vi "WLAN Two Site Example_Remote PC.vi"(5 "Single DUT Mode?":bool, 7 "Stop if fail":bool, 9 "Select Test Item (TX Verification)":T1={"Tx_ 802.11a/g OFDM"=TRUE, "Tx_ 802.11b DSSS/CCK"=FALSE, "Tx_ 802.11n OFDM "=TRUE, "Tx_ 802.11ac OFDM "=TRUE}, 10 "Select Test Content":T3, 11 "SET RUN TIMES":i32=1) -> (1 "Results":T2, 2 "Total test time":dbl=137.063, 3 "RUN TIMES":i32=1)   [LabVIEW 2012]
uses:
  WLAN SubVIs/WLAN Autotest Library/niWLAN/WLAN -  niWLAN - INC - Select Measurement.ctl
  System SubVIs/Select_Test_Content.ctl
  Report SubVIs/TypeDef/Report Log Flow Control.ctl
  Report SubVIs/TypeDef/DUT Number.ctl
  WLAN SubVIs/WLAN Autotest Library/TestExample/QCA/WB335B/TypeDef/WLAN Flow Control.ctl
  System SubVIs/Ctl_Ant_Number.ctl
  Remote Sever SubVIs/TypeDef/Send Command Message.ctl
panel:
  in  "Select Test Item (TX Verification) 2":T1={"Tx_ 802.11a/g OFDM"=TRUE, "Tx_ 802.11b DSSS/CCK"=FALSE, "Tx_ 802.11n OFDM "=TRUE, "Tx_ 802.11ac OFDM "=TRUE}
  out "RUN TIMES 2":i32=1
  out "MAC&SN 3":string
  out "Results 2":T2
  out "MAC&SN 2":string
  out "MAC&SN":string
  out "DUT2 log path":path
  out "DUT1 log path":path
  in  "Tab Control":T4(tab)
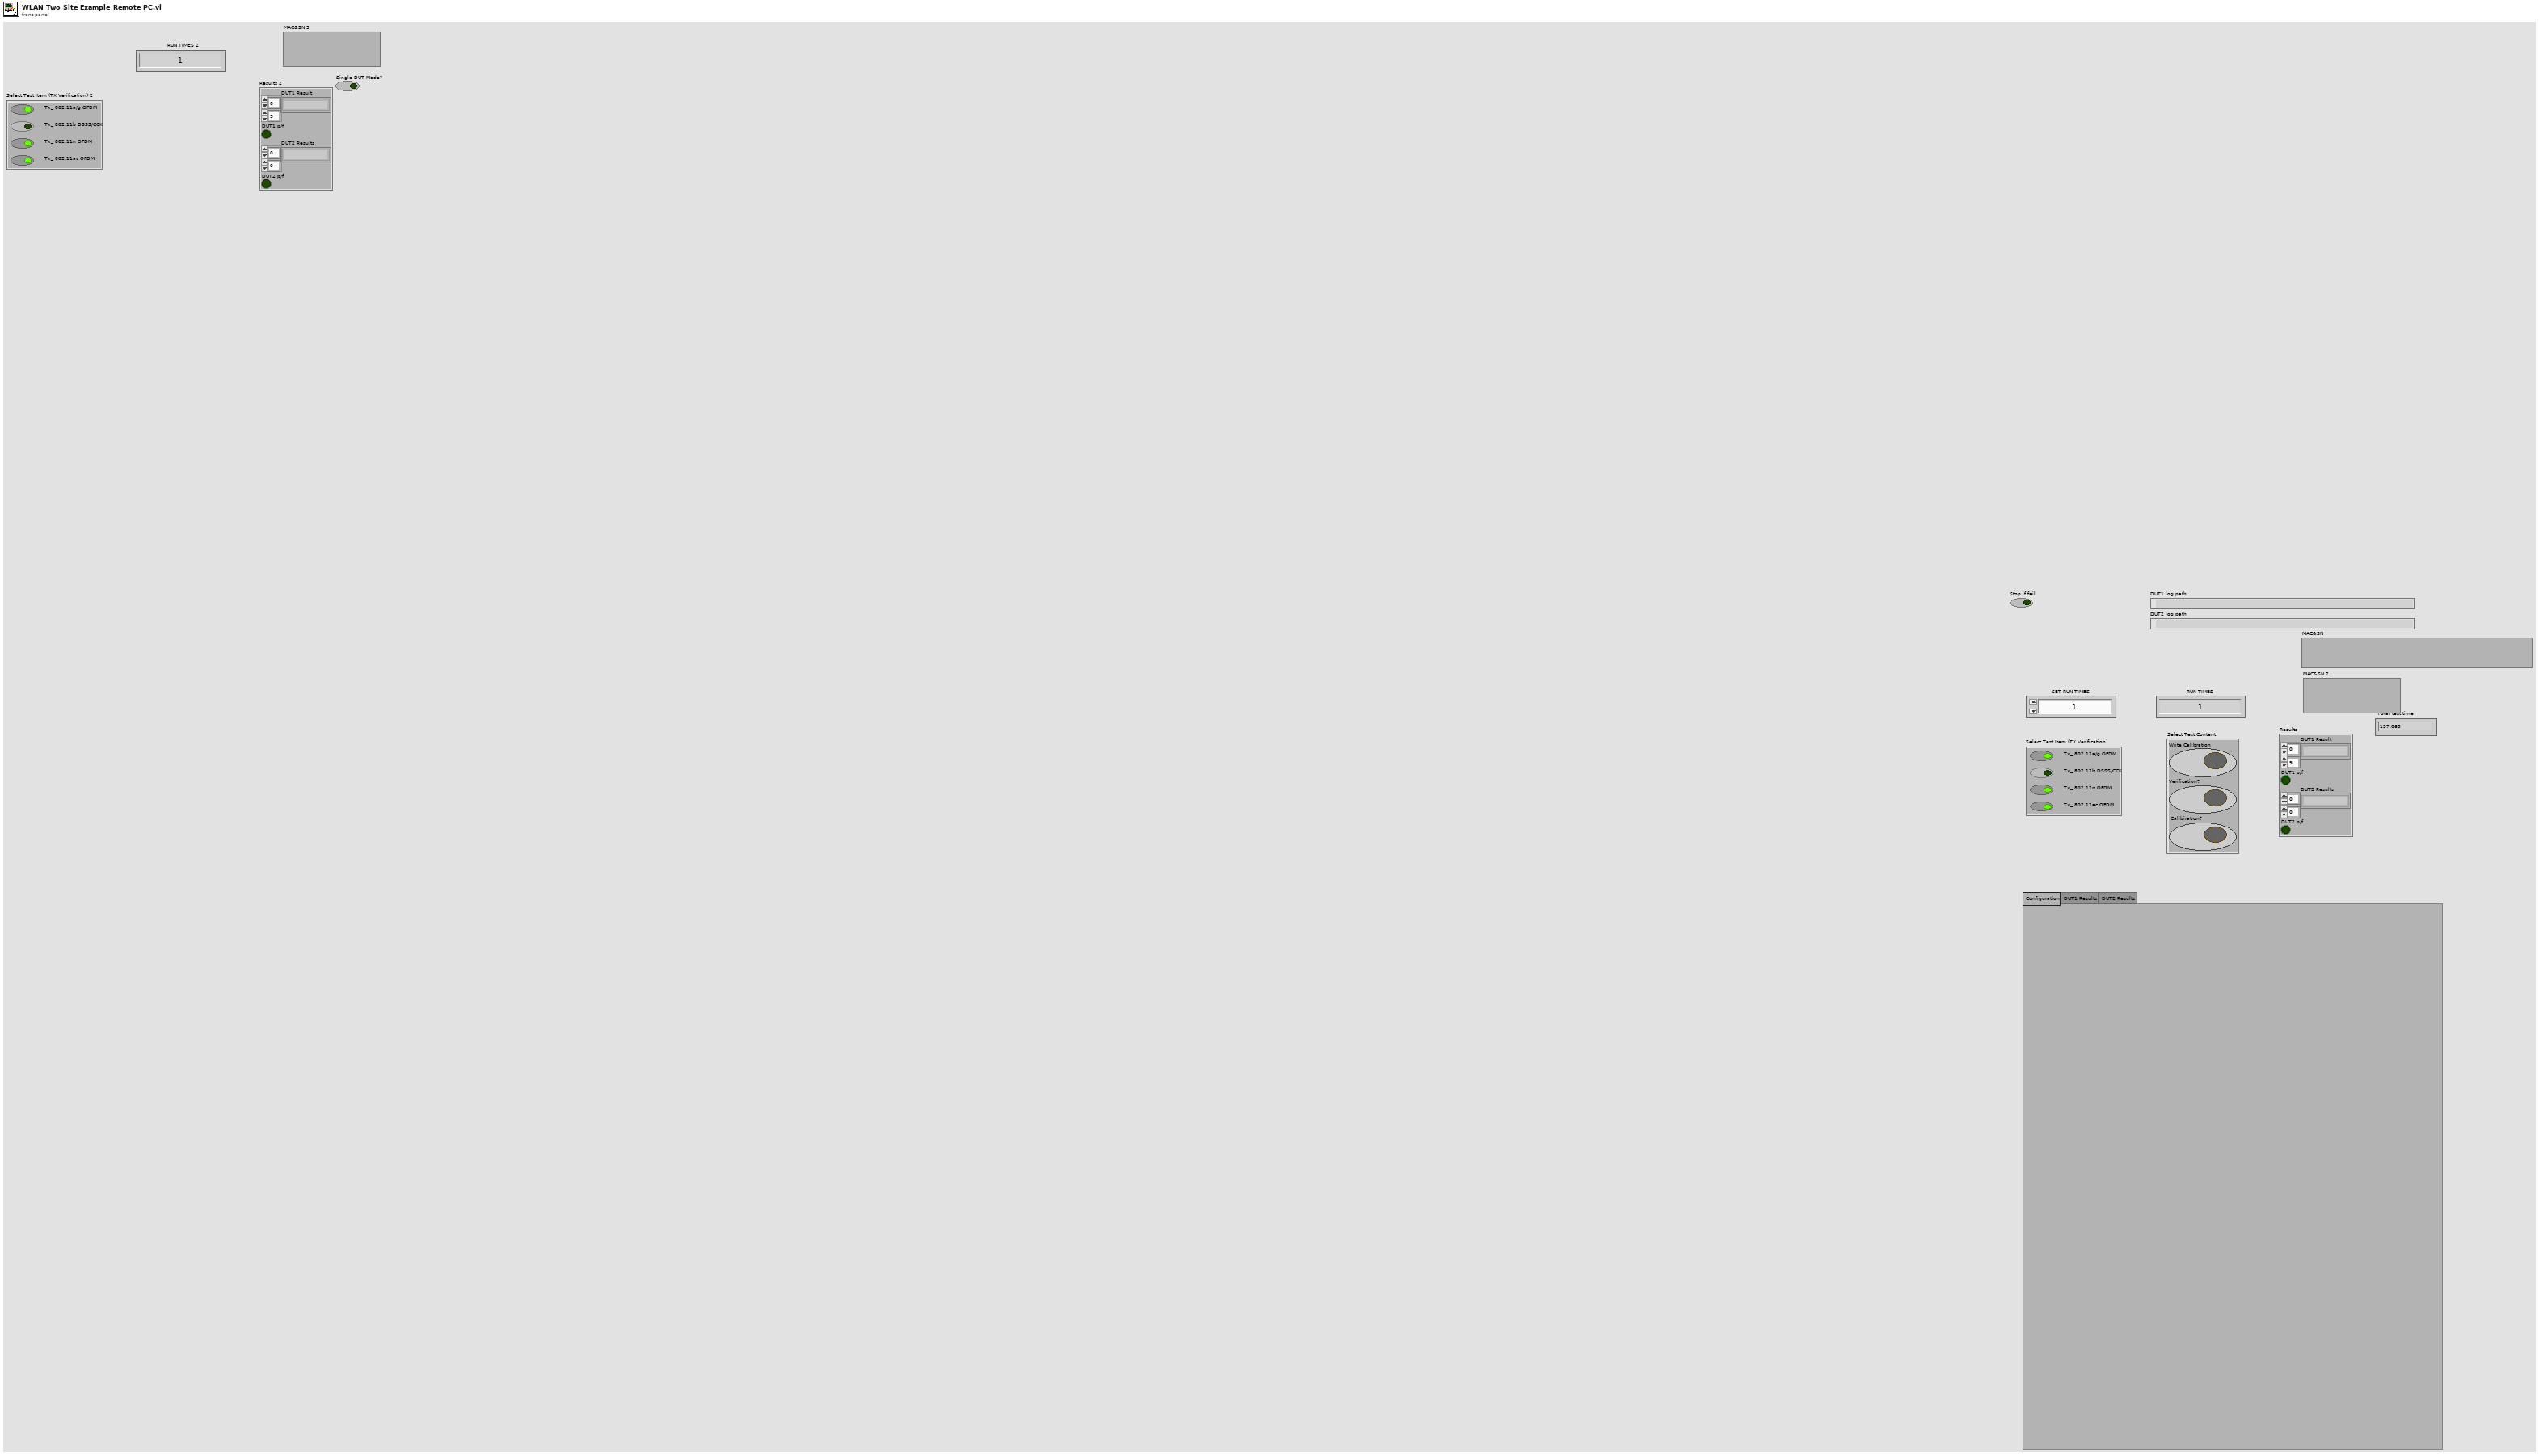
[diagram p1: front panel]
types:
  T1 = typedef "WLAN -  niWLAN - INC - Select Measurement.ctl" = cluster{"Tx_ 802.11a/g OFDM":bool, "Tx_ 802.11b DSSS/CCK":bool, "Tx_ 802.11n OFDM ":bool, "Tx_ 802.11ac OFDM ":bool}
  T2 = cluster{"DUT1 Result":string[][], "DUT1 p/f":bool, "DUT2 Results":string[][], "DUT2 p/f":bool}
  T3 = typedef "Select_Test_Content.ctl" = cluster{"Write Calibration":bool, "Verification?":bool, " Calibiration?":bool}
  T4 = enum32{"Configuration", "DUT1 Results", "DUT2 Results "}
  T5 = typedef "DUT Number.ctl" = string
  T6 = typedef "Report Log Flow Control.ctl" = enum16{"Create Log File", "Append Test Item Head", "Append WLAN TX IQ Result", "Append WLAN TX Spectrum Result", "Append WLAN RX Result", "Append BT TX BR Result", "Append BT TX EDR Result", "Append Customized Text", "Append BT RX Result", "Read Log File", "Save Test Time"}
  T7 = typedef "WLAN Flow Control.ctl" = enum16{"Initial WLAN DUT", "Load WLAN DUT Only", "Close WLAN Test", "Power Calibration", "TX Verification", "RX Verification", "Write Memory"}
  T8 = typedef "Send Command Message.ctl" = string
  T9 = typedef "Ctl_Ant_Number.ctl" = enum16{"1", "2", "3"}
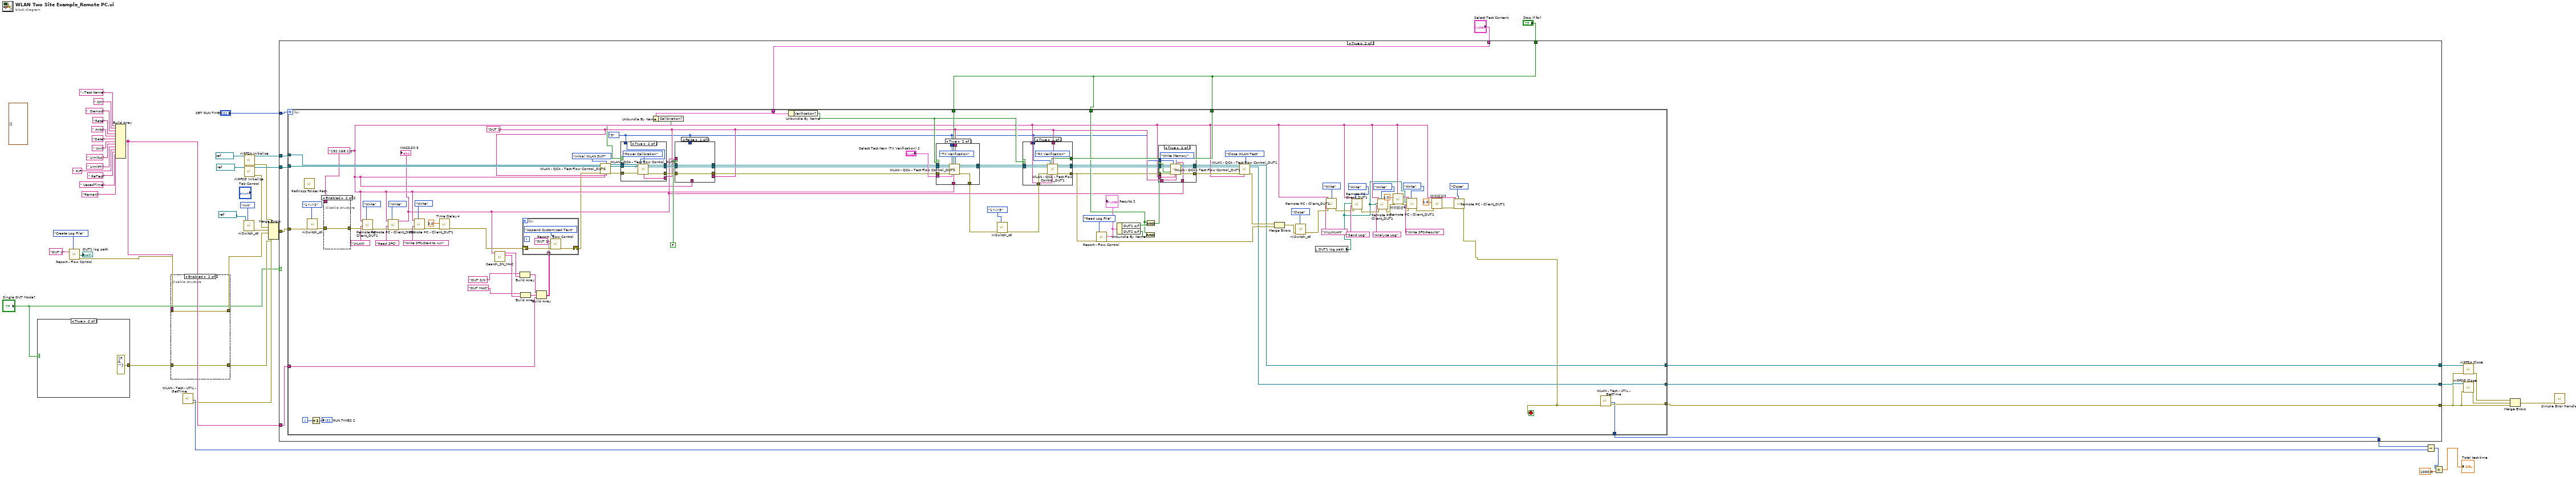
[diagram p0: block diagram]
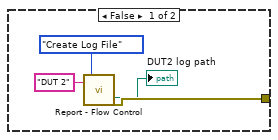
[diagram p2: hidden frame]
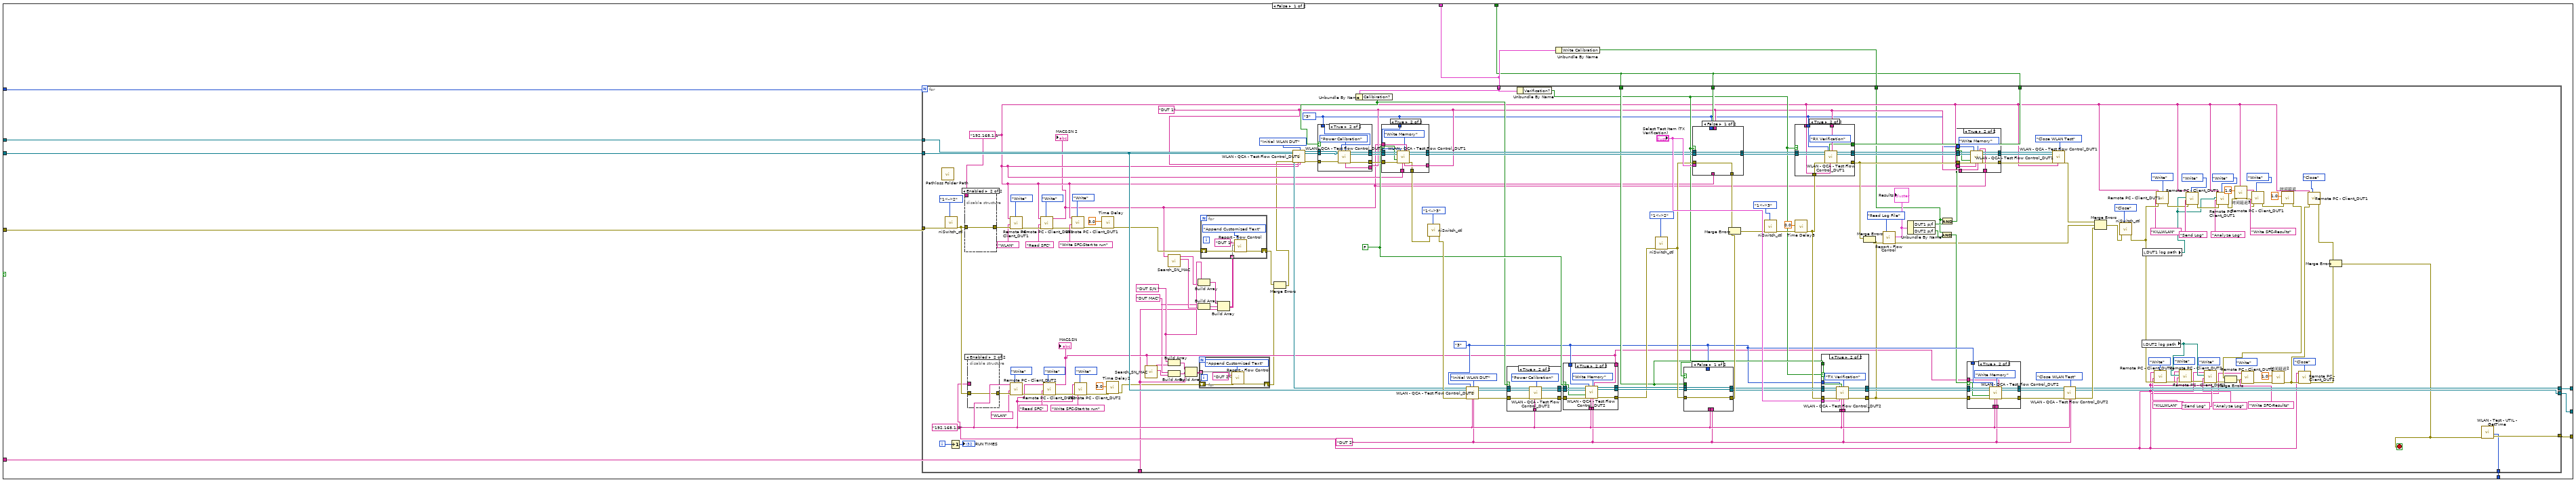
[diagram p3: hidden frame]
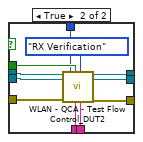
[diagram p7: hidden frame]
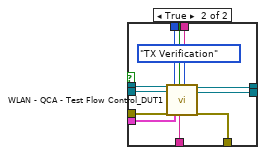
[diagram p10: hidden frame]
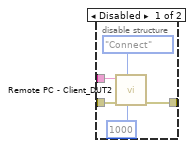
[diagram p12: hidden frame]
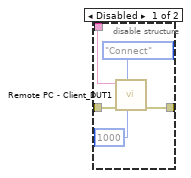
[diagram p13: hidden frame]
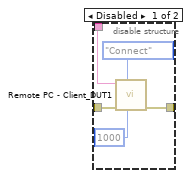
[diagram p20: hidden frame]
diagram:
  (unwired) cluster{u32, u32, u32, u32, u32, u32}[] [] ("History Data")
  n1 = case shown="True" "Single DUT Mode?" {
    tunnel: [w49 errorcluster {"status"=FALSE, "code"=0, "source"=""} ("error out")] -> w19
    frame False {
      n2 = call "Report - Flow Control.vi"("DUT Number (Each Control)"=T5 "DUT 2", "Reprot Log Flow Control"=Report_Log_Flow_Control."Create Log File") -> ("DUT2 log path"=→"DUT2 log path":path, "error out"=w49:errorcluster)  [unwired: 12 in, 4 out]
    }
    frame True {
    }
  }
  n3 = call "Report - Flow Control.vi"("DUT Number (Each Control)"=T5 "DUT 1", "Reprot Log Flow Control"=Report_Log_Flow_Control."Create Log File") -> ("DUT1 log path"=→"DUT1 log path":path, "error out"=w20:errorcluster)  [unwired: 12 in, 4 out]
  n4 = Build Array(";;Test Name", " CH", "  Demod", "Rate", " Ants", "Data", " Unit", " LimitLo", " LimitHi", " P/F", " ReTest", " UesedTime", "Remark" ("元素")) -> (w6:string[])
  n5 = disable-structure shown="Enabled" {
    disable-tunnel: [w57 w62] -> w27
    disable-tunnel: [w56 w63] -> w26
    disable-tunnel: w20 -> [w55 w63]
    disable-tunnel: w19 -> [w54 w62]
    disable-tunnel: w6 -> [w53 _]
    frame Disabled {
      n6 = call "Report - Flow Control.vi"("DUT Number (Each Control)"=T5 "DUT 1", "Text Input"=w53, "error in"=w55, "Reprot Log Flow Control"=Report_Log_Flow_Control."Append Customized Text") -> ("error out"=w56:errorcluster)  [unwired: 10 in, 5 out]
      n7 = call "Report - Flow Control.vi"("DUT Number (Each Control)"=T5 "DUT 2", "Text Input"=w53, "error in"=w54, "Reprot Log Flow Control"=Report_Log_Flow_Control."Append Customized Text") -> ("error out"=w57:errorcluster)  [unwired: 10 in, 5 out]
    }
    frame Enabled {
    }
  }
  n8 = call "WLAN - Test - UTIL - GetTime.vi"() -> ("error out"=w31:errorcluster, "millisecond timer value"=w32:u32)  [unwired: 9 in, 1 out]
  n9 = call "niSwitch_ctl.vi"("Flow Control"=enum16{"Init", "1<->2", "1<->3", "Close"}."Init" ("Ctrl"), "Switch In"=refnum<k15> "2598" ("resource name")) -> ("error out"=w40:errorcluster)  [unwired: 7 in, 2 out]
  n10 = call <instrlib>:"niRFSA Initialize.vi"("resource name"=refnum<k15> "VST1") -> ("instrument handle"=w45:refnum<k15>, "error out"=w42:errorcluster)  [unwired: 13 in]
  n11 = call <instrlib>:"niRFSG Initialize.vi"("resource name"=refnum<k15> "VST1") -> ("instrument handle"=w44:refnum<k15>, "error out"=w41:errorcluster)  [unwired: 13 in]
  n12 = Merge Errors(w42, w41, w40, w26, w27, w31) -> (w39:errorcluster)
  n13 = case shown="True" "Single DUT Mode?" {
    tunnel: w45 -> [w75 w413]
    tunnel: w44 -> [w74 w412]
    tunnel: "SET RUN TIMES" -> [w73 w411]
    tunnel: w39 -> [w72 w414]
    tunnel: [w71 w406] -> w2
    tunnel: [w70 w405] -> w36
    tunnel: [w69 w407] -> w35
    tunnel: w6 -> [w68 w410]
    tunnel: [w67 w404] -> w5
    tunnel: "Select Test Content" -> [w65 w409]
    tunnel: "Stop if fail" -> [w64 w408]
    frame False {
      n14 = Unbundle By Name(w65) -> ("Write Calibration"=w66:bool)
      n15 = for {
        N: w73 -> [_]
        tunnel: w72 -> [w237]
        tunnel: w75 -> [w179]
        tunnel: w74 -> [w224]
        tunnel: [w193] -> w67
        tunnel: [w207] -> w71
        tunnel: [w206] -> w70
        tunnel: [w192] -> w69
        tunnel: w64 -> [w143]
        tunnel: w64 -> [w129]
        tunnel: w64 -> [w142]
        tunnel: w65 -> [w128]
        tunnel: w66 -> [w111]
        tunnel: w68 -> [w83]
        i -> [w234]
        stop <- w194 stop-if-true
        w88 = "DUT MAC" ("string")
        w89 = "DUT S/N " ("string")
        w130 = FALSE
        (unwired) enum16{"Connect", "Read", "Write", "Close"}."Write" ("Flow Contorl")
        (unwired) enum16{"Connect", "Read", "Write", "Close"}."Write" ("Flow Contorl")
        (unwired) enum16{"Connect", "Read", "Write", "Close"}."Write" ("Flow Contorl")
        w101 = Ctl_Ant_Number."3" ("Ant Number")
        w108 = Ctl_Ant_Number."3" ("Ant Number")
        w103 = "192.168.1.2" ("ART2 IP Address (\"\": localhost) (Initial)")
        w102 = "DUT 2" ("Board Name (TX RX Verification)")
        w113 = "DUT 1" ("Board Name (TX RX Verification)")
        w114 = "192.168.1.1" ("ART2 IP Address (\"\": localhost)")
        n16 = call "Pathloss Folder Path.vi"() -> ()  [unwired: 11 in, 1 out]
        n17 = call "niSwitch_ctl.vi"("Flow Control"=enum16{"Init", "1<->2", "1<->3", "Close"}."1<->2", "error in"=w237) -> ("error out"=w170:errorcluster)  [unwired: 7 in, 2 out]
        n18 = Increment(x=w234) -> (x+1=→"RUN TIMES":i32)
        n19 = disable-structure shown="Enabled" {
          disable-tunnel: [w371 w373] -> w232
          disable-tunnel: w170 -> [w369 w373]
          disable-tunnel: w114 -> [w368 _]
          frame Disabled {
            n20 = call "Remote PC - Client_DUT1.vi"("Remote Sever Port (2800)"=u16 1000, "Flow Contorl"=enum16{"Connect", "Read", "Write", "Close"}."Connect", "error in"=w369, "IP Address"=w368) -> ("error out"=w371:errorcluster)  [unwired: 5 in, 2 out]
          }
          frame Enabled {
          }
        }
        n21 = disable-structure shown="Enabled" {
          disable-tunnel: [w365 w367] -> w219
          disable-tunnel: w170 -> [w363 w367]
          disable-tunnel: w103 -> [w362 _]
          frame Disabled {
            n22 = call "Remote PC - Client_DUT2.vi"("Remote Sever Port (2800)"=u16 1000, "Flow Contorl"=enum16{"Connect", "Read", "Write", "Close"}."Connect", "error in"=w363, "IP Address"=w362) -> ("error out"=w365:errorcluster)  [unwired: 5 in, 2 out]
          }
          frame Enabled {
          }
        }
        n23 = call "Remote PC - Client_DUT2.vi"("Flow Contorl"=enum16{"Connect", "Read", "Write", "Close"}."Write", "error in"=w219, "Send Command"=T8 "WLAN", "IP Address"=w103) -> ("error out"=w177:errorcluster)  [unwired: 5 in, 2 out]
        n24 = call "Remote PC - Client_DUT1.vi"("Flow Contorl"=enum16{"Connect", "Read", "Write", "Close"}."Write", "error in"=w232, "Send Command"=T8 "WLAN", "IP Address"=w114) -> ("error out"=w166:errorcluster)  [unwired: 5 in, 2 out]
        n25 = call "Remote PC - Client_DUT1.vi"("Flow Contorl"=enum16{"Connect", "Read", "Write", "Close"}."Write", "error in"=w166, "Send Command"=T8 "Read SFC", "IP Address"=w114) -> ("error out"=w163:errorcluster, "MAC&SN"=w96:string)  [unwired: 5 in, 1 out]
        "MAC&SN 2" <- w96
        n26 = call "Remote PC - Client_DUT2.vi"("Flow Contorl"=enum16{"Connect", "Read", "Write", "Close"}."Write", "error in"=w177, "Send Command"=T8 "Read SFC", "IP Address"=w103) -> ("error out"=w173:errorcluster, "MAC&SN"=w90:string)  [unwired: 5 in, 1 out]
        "MAC&SN" <- w90
        n27 = call "Remote PC - Client_DUT1.vi"("Flow Contorl"=enum16{"Connect", "Read", "Write", "Close"}."Write", "error in"=w163, "Send Command"=T8 "Write SFC-Start to run", "IP Address"=w114) -> ("error out"=w162:errorcluster)  [unwired: 5 in, 2 out]
        n28 = call "Remote PC - Client_DUT2.vi"("Flow Contorl"=enum16{"Connect", "Read", "Write", "Close"}."Write", "error in"=w173, "Send Command"=T8 "Write SFC-Start to run", "IP Address"=w103) -> ("error out"=w172:errorcluster)  [unwired: 5 in, 2 out]
        n29 = call "Time Delay"("error in (no error)"=w162, "Delay Time (s)"=3.0) -> ("error out"=w97:errorcluster)  [unwired: 9 in]
        n30 = call "Time Delay2"("error in (no error)"=w172, "Delay Time (s)"=3.0) -> ("error out"=w81:errorcluster)  [unwired: 9 in]
        n31 = call "Search_SN_MAC.vi"("MAC&SN"=w90) -> ("MAC"=w86:string, "SN"=w87:string)  [unwired: 9 in]
        n32 = call "Search_SN_MAC.vi"("MAC&SN"=w96) -> ("MAC"=w94:string, "SN"=w95:string)  [unwired: 9 in]
        n33 = Build Array(w89, w87) -> (w85:string[])
        n34 = Build Array(w88, w86) -> (w84:string[])
        n35 = Build Array(w85, w84, w83) -> (w82:string[][])
        n36 = Build Array(w89, w95) -> (w93:string[])
        n37 = Build Array(w88, w94) -> (w92:string[])
        n38 = for {
          tunnel: w82 -> [w243] mode=indexing
          shift-right: [w241] -> w79
          shift-left: w81 -> [w242]
          n39 = call "Report - Flow Control.vi"("DUT Number (Each Control)"=T5 "DUT 2", "Text Input"=w243, "error in"=w242, "Reprot Log Flow Control"=Report_Log_Flow_Control."Append Customized Text") -> ("error out"=w241:errorcluster)  [unwired: 10 in, 5 out]
        }
        n40 = Build Array(w93, w92, w83) -> (w91:string[][])
        n41 = for {
          shift-right: [w247] -> w80
          shift-left: w97 -> [w248]
          tunnel: w91 -> [w246] mode=indexing
          n42 = call "Report - Flow Control.vi"("DUT Number (Each Control)"=T5 "DUT 1", "Text Input"=w246, "error in"=w248, "Reprot Log Flow Control"=Report_Log_Flow_Control."Append Customized Text") -> ("error out"=w247:errorcluster)  [unwired: 10 in, 5 out]
        }
        n43 = Merge Errors(w80, w79) -> (w78:errorcluster)
        n44 = call "WLAN - QCA - Test Flow Control_DUT1.vi"("RFSA In (Initial)"=w179, "RFSG In (Initial)"=w224, "error in"=w78, "NB IP (Initial)"=w114, "Function"=WLAN_Flow_Control."Initial WLAN DUT", "DUT Number (Initial, Create Log, Save Time)"=w113) -> ("RFSA Out"=w212:refnum<k15>, "RFSG Out"=w211:refnum<k15>, "error out"=w236:errorcluster)  [unwired: 10 in, 1 out]
        n45 = Unbundle By Name(w128) -> ("Calibiration?"=w127:bool)
        n46 = case shown="True" w127 {
          tunnel: w236 -> [w350 w361]
          tunnel: w212 -> [w352 w360]
          tunnel: w211 -> [w351 w359]
          tunnel: [w352 w358] -> w191
          tunnel: [w351 w357] -> w190
          tunnel: [w350 w356] -> w187
          tunnel: w113 -> [_ w355]
          tunnel: w108 -> [_ w354]
          frame False {
          }
          frame True {
            n47 = call "WLAN - QCA - Test Flow Control_DUT1.vi"("RFSA In (Initial)"=w360, "RFSG In (Initial)"=w359, "error in"=w361, "Ant Number"=w354, "Function"=WLAN_Flow_Control."Power Calibration", "DUT Number (Initial, Create Log, Save Time)"=w355) -> ("RFSA Out"=w358:refnum<k15>, "RFSG Out"=w357:refnum<k15>, "error out"=w356:errorcluster)  [unwired: 10 in, 1 out]
          }
        }
        n48 = case shown="True" w130 {
          selector: w130 -> [_ w392]
          tunnel: w191 -> [w391 w403]
          tunnel: w190 -> [w390 w402]
          tunnel: [w391 w401] -> w189
          tunnel: [w390 w400] -> w188
          tunnel: w113 -> [_ w399]
          tunnel: w187 -> [w389 w398]
          tunnel: [w389 w397] -> w186
          tunnel: w108 -> [_ w396]
          tunnel: w114 -> [_ w395]
          tunnel: w96 -> [_ w394]
          frame False {
          }
          frame True {
            n49 = call "WLAN - QCA - Test Flow Control_DUT1.vi"("RFSA In (Initial)"=w403, "RFSG In (Initial)"=w402, "Write Calibration"=w392, "error in"=w398, "Ant Number"=w396, "NB IP (Initial)"=w395, "Function"=WLAN_Flow_Control."Write Memory", "DUT Number (Initial, Create Log, Save Time)"=w399, "MAC&SN"=w394) -> ("RFSA Out"=w401:refnum<k15>, "RFSG Out"=w400:refnum<k15>, "error out"=w397:errorcluster)  [unwired: 7 in, 1 out]
          }
        }
        n50 = call "niSwitch_ctl.vi"("Flow Control"=enum16{"Init", "1<->2", "1<->3", "Close"}."1<->3", "error in"=w186) -> ("error out"=w203:errorcluster)  [unwired: 7 in, 2 out]
        n51 = call "WLAN - QCA - Test Flow Control_DUT2.vi"("RFSA In (Initial)"=w179, "RFSG In (Initial)"=w224, "error in"=w203, "Ant Number"=w101, "NB IP (Initial)"=w103, "Function"=WLAN_Flow_Control."Initial WLAN DUT", "DUT Number (Initial, Create Log, Save Time)"=w102) -> ("RFSA Out"=w223:refnum<k15>, "RFSG Out"=w222:refnum<k15>, "error out"=w225:errorcluster)  [unwired: 9 in, 1 out]
        n52 = case shown="True" w127 {
          tunnel: w225 -> [w310 w320]
          tunnel: w223 -> [w312 w319]
          tunnel: w222 -> [w311 w318]
          tunnel: [w312 w317] -> w185
          tunnel: [w311 w316] -> w184
          tunnel: [w310 w315] -> w181
          tunnel: w103 -> [_ w314]
          frame False {
          }
          frame True {
            n53 = call "WLAN - QCA - Test Flow Control_DUT2.vi"("RFSA In (Initial)"=w319, "RFSG In (Initial)"=w318, "error in"=w320, "NB IP (Initial)"=w314, "Function"=WLAN_Flow_Control."Power Calibration") -> ("RFSA Out"=w317:refnum<k15>, "RFSG Out"=w316:refnum<k15>, "error out"=w315:errorcluster)  [unwired: 11 in, 1 out]
          }
        }
        n54 = Unbundle By Name(w128) -> ("Verification?"=w126:bool)
        n55 = case shown="True" w130 {
          selector: w130 -> [_ w377]
          tunnel: w185 -> [w376 w388]
          tunnel: w184 -> [w375 w387]
          tunnel: [w376 w386] -> w183
          tunnel: [w375 w385] -> w182
          tunnel: w101 -> [_ w384]
          tunnel: w181 -> [w374 w383]
          tunnel: [w374 w382] -> w180
          tunnel: w102 -> [_ w381]
          tunnel: w103 -> [_ w380]
          tunnel: w90 -> [_ w379]
          frame False {
          }
          frame True {
            n56 = call "WLAN - QCA - Test Flow Control_DUT2.vi"("RFSA In (Initial)"=w388, "RFSG In (Initial)"=w387, "Write Calibration"=w377, "error in"=w383, "Ant Number"=w384, "NB IP (Initial)"=w380, "Function"=WLAN_Flow_Control."Write Memory", "DUT Number (Initial, Create Log, Save Time)"=w381, "MAC&SN"=w379) -> ("RFSA Out"=w386:refnum<k15>, "RFSG Out"=w385:refnum<k15>, "error out"=w382:errorcluster)  [unwired: 7 in, 1 out]
          }
        }
        n57 = call "niSwitch_ctl.vi"("Flow Control"=enum16{"Init", "1<->2", "1<->3", "Close"}."1<->2", "error in"=w180) -> ("error out"=w201:errorcluster)  [unwired: 7 in, 2 out]
        n58 = case shown="False" w126 {
          tunnel: [w296 w309] -> w220
          tunnel: [w298 w308] -> w214
          tunnel: [w297 w307] -> w213
          tunnel: w201 -> [w296 w306]
          tunnel: w183 -> [w298 w305]
          tunnel: w182 -> [w297 w304]
          tunnel: w142 -> [_ w303]
          tunnel: w103 -> [_ w302]
          tunnel: w102 -> [_ w301]
          tunnel: w101 -> [_ w300]
          frame False {
          }
          frame True {
            n59 = call "WLAN - QCA - Test Flow Control_DUT2.vi"("RFSA In (Initial)"=w305, "RFSG In (Initial)"=w304, "error in"=w306, "Ant Number"=w300, "Stop if fail"=w303, "NB IP (Initial)"=w302, "Function"=WLAN_Flow_Control."RX Verification", "DUT Number (Initial, Create Log, Save Time)"=w301) -> ("RFSA Out"=w308:refnum<k15>, "RFSG Out"=w307:refnum<k15>, "error out"=w309:errorcluster)  [unwired: 8 in, 1 out]
          }
        }
        n60 = case shown="False" w126 {
          tunnel: "Select Test Item (TX Verification)" -> [_ w348]
          tunnel: [w337 w347] -> w221
          tunnel: [w336 w346] -> w210
          tunnel: [w335 w345] -> w209
          tunnel: w201 -> [w337 w344]
          tunnel: w189 -> [w336 w343]
          tunnel: w188 -> [w335 w342]
          tunnel: w143 -> [_ w341]
          tunnel: w114 -> [_ w340]
          tunnel: w113 -> [_ w339]
          tunnel: w108 -> [_ w338]
          frame False {
          }
          frame True {
            n61 = call "WLAN - QCA - Test Flow Control_DUT1.vi"("RFSA In (Initial)"=w343, "RFSG In (Initial)"=w342, "error in"=w344, "Ant Number"=w338, "Select Test Item (TX Verification)"=w348, "Stop if fail"=w341, "NB IP (Initial)"=w340, "Function"=WLAN_Flow_Control."TX Verification", "DUT Number (Initial, Create Log, Save Time)"=w339) -> ("RFSA Out"=w346:refnum<k15>, "RFSG Out"=w345:refnum<k15>, "error out"=w347:errorcluster)  [unwired: 7 in, 1 out]
          }
        }
        n62 = Merge Errors(w221, w220) -> (w205:errorcluster)
        n63 = call "niSwitch_ctl.vi"("Flow Control"=enum16{"Init", "1<->2", "1<->3", "Close"}."1<->3", "error in"=w205) -> ("error out"=w197:errorcluster)  [unwired: 7 in, 2 out]
        n64 = call "Time Delay3"("error in (no error)"=w197, "Delay Time (s)"=0.0) -> ("error out"=w196:errorcluster)  [unwired: 9 in]
        n65 = case shown="True" w126 {
          tunnel: [w321 w334] -> w116
          tunnel: w210 -> [w323 w333]
          tunnel: w209 -> [w322 w332]
          tunnel: [w323 w331] -> w120
          tunnel: [w322 w330] -> w119
          tunnel: w196 -> [w321 w329]
          tunnel: w114 -> [_ w328]
          tunnel: w113 -> [_ w327]
          tunnel: w108 -> [_ w326]
          tunnel: w129 -> [_ w324]
          frame False {
          }
          frame True {
            n66 = call "WLAN - QCA - Test Flow Control_DUT1.vi"("RFSA In (Initial)"=w333, "RFSG In (Initial)"=w332, "error in"=w329, "Ant Number"=w326, "Stop if fail"=w324, "NB IP (Initial)"=w328, "Function"=WLAN_Flow_Control."RX Verification", "DUT Number (Initial, Create Log, Save Time)"=w327) -> ("RFSA Out"=w331:refnum<k15>, "RFSG Out"=w330:refnum<k15>, "error out"=w334:errorcluster)  [unwired: 8 in, 1 out]
          }
        }
        n67 = case shown="True" w126 {
          tunnel: "Select Test Item (TX Verification)" -> [_ w294]
          tunnel: [w281 w293] -> w99
          tunnel: w214 -> [w283 w292]
          tunnel: w213 -> [w282 w291]
          tunnel: [w283 w290] -> w107
          tunnel: [w282 w289] -> w105
          tunnel: w196 -> [w281 w288]
          tunnel: w142 -> [_ w287]
          tunnel: w103 -> [_ w286]
          tunnel: w102 -> [_ w285]
          tunnel: w101 -> [_ w284]
          frame False {
          }
          frame True {
            n68 = call "WLAN - QCA - Test Flow Control_DUT2.vi"("RFSA In (Initial)"=w292, "RFSG In (Initial)"=w291, "error in"=w288, "Ant Number"=w284, "Select Test Item (TX Verification)"=w294, "Stop if fail"=w287, "NB IP (Initial)"=w286, "Function"=WLAN_Flow_Control."TX Verification", "DUT Number (Initial, Create Log, Save Time)"=w285) -> ("RFSA Out"=w290:refnum<k15>, "RFSG Out"=w289:refnum<k15>, "error out"=w293:errorcluster)  [unwired: 7 in, 1 out]
          }
        }
        n69 = Merge Errors(w116, w99) -> (w121:errorcluster)
        n70 = call "Report - Flow Control.vi"("error in"=w121, "Reprot Log Flow Control"=Report_Log_Flow_Control."Read Log File") -> ("Cluster 2"=w123:T2, "error out"=w76:errorcluster)  [unwired: 12 in, 4 out]
        "Results" <- w123
        n71 = Unbundle By Name(w123) -> ("DUT1 p/f"=w112:bool, "DUT2 p/f"=w110:bool)
        n72 = And(x=w111, y=w110) -> (x .and. y?=w100:bool)
        n73 = And(x=w111, y=w112) -> (x .and. y?=w109:bool)
        n74 = case shown="True" w109 {
          selector: w109 -> [_ w271]
          tunnel: w120 -> [w268 w280]
          tunnel: w119 -> [w267 w279]
          tunnel: [w268 w278] -> w118
          tunnel: [w267 w277] -> w117
          tunnel: w116 -> [w266 w276]
          tunnel: [w266 w275] -> w115
          tunnel: w114 -> [_ w274]
          tunnel: w113 -> [_ w273]
          tunnel: w108 -> [_ w270]
          tunnel: w96 -> [_ w269]
          frame False {
          }
          frame True {
            n75 = call "WLAN - QCA - Test Flow Control_DUT1.vi"("RFSA In (Initial)"=w280, "RFSG In (Initial)"=w279, "Write Calibration"=w271, "error in"=w276, "Ant Number"=w270, "NB IP (Initial)"=w274, "Function"=WLAN_Flow_Control."Write Memory", "DUT Number (Initial, Create Log, Save Time)"=w273, "MAC&SN"=w269) -> ("RFSA Out"=w278:refnum<k15>, "RFSG Out"=w277:refnum<k15>, "error out"=w275:errorcluster)  [unwired: 7 in, 1 out]
          }
        }
        n76 = case shown="True" w100 {
          selector: w100 -> [_ w256]
          tunnel: w107 -> [w253 w265]
          tunnel: [w253 w264] -> w106
          tunnel: w105 -> [w252 w263]
          tunnel: [w252 w262] -> w104
          tunnel: w103 -> [_ w261]
          tunnel: w102 -> [_ w260]
          tunnel: w101 -> [_ w258]
          tunnel: w90 -> [_ w257]
          tunnel: w99 -> [w251 w255]
          tunnel: [w251 w254] -> w98
          frame False {
          }
          frame True {
            n77 = call "WLAN - QCA - Test Flow Control_DUT2.vi"("RFSA In (Initial)"=w265, "RFSG In (Initial)"=w263, "Write Calibration"=w256, "error in"=w255, "Ant Number"=w258, "NB IP (Initial)"=w261, "Function"=WLAN_Flow_Control."Write Memory", "DUT Number (Initial, Create Log, Save Time)"=w260, "MAC&SN"=w257) -> ("RFSA Out"=w264:refnum<k15>, "RFSG Out"=w262:refnum<k15>, "error out"=w254:errorcluster)  [unwired: 7 in, 1 out]
          }
        }
        n78 = call "WLAN - QCA - Test Flow Control_DUT1.vi"("RFSA In (Initial)"=w118, "RFSG In (Initial)"=w117, "error in"=w115, "NB IP (Initial)"=w114, "Function"=WLAN_Flow_Control."Close WLAN Test") -> ("error out"=w77:errorcluster)  [unwired: 11 in, 3 out]
        n79 = call "WLAN - QCA - Test Flow Control_DUT2.vi"("RFSA In (Initial)"=w106, "RFSG In (Initial)"=w104, "error in"=w98, "NB IP (Initial)"=w103, "Function"=WLAN_Flow_Control."Close WLAN Test", "DUT Number (Initial, Create Log, Save Time)"=w102) -> ("RFSA Out"=w207:refnum<k15>, "RFSG Out"=w206:refnum<k15>, "error out"=w216:errorcluster)  [unwired: 10 in, 1 out]
        n80 = Merge Errors(w77, w76, w216) -> (w199:errorcluster)
        n81 = call "niSwitch_ctl.vi"("Flow Control"=enum16{"Init", "1<->2", "1<->3", "Close"}."Close", "error in"=w199) -> ("error out"=w198:errorcluster)  [unwired: 7 in, 2 out]
        n82 = local read "DUT2 log path"() -> (w146:path)
        n83 = local read "DUT1 log path"() -> (w147:path)
        n84 = call "Remote PC - Client_DUT2.vi"("Flow Contorl"=enum16{"Connect", "Read", "Write", "Close"}."Write", "error in"=w198, "Send Command"=T8 "KILLWLAN", "IP Address"=w103) -> ("error out"=w145:errorcluster)  [unwired: 5 in, 2 out]
        n85 = call "Remote PC - Client_DUT1.vi"("Flow Contorl"=enum16{"Connect", "Read", "Write", "Close"}."Write", "error in"=w198, "Send Command"=T8 "KILLWLAN", "IP Address"=w114) -> ("error out"=w158:errorcluster)  [unwired: 5 in, 2 out]
        n86 = call "Remote PC - Client_DUT2.vi"("error in"=w145, "Send Command"=T8 "Send Log", "Log Path"=w146, "IP Address"=w103) -> ("error out"=w144:errorcluster)  [unwired: 5 in, 2 out]
        n87 = call "Remote PC - Client_DUT1.vi"("Flow Contorl"=enum16{"Connect", "Read", "Write", "Close"}."Write", "error in"=w158, "Send Command"=T8 "Send Log", "Log Path"=w147, "IP Address"=w114) -> ("error out"=w157:errorcluster)  [unwired: 4 in, 2 out]
        n88 = call "Remote PC - Client_DUT2.vi"("error in"=w144, "Send Command"=T8 "Analyze Log", "Log Path"=w146, "IP Address"=w103) -> ("error out"=w134:errorcluster)  [unwired: 5 in, 2 out]
        n89 = call "Remote PC - Client_DUT1.vi"("Flow Contorl"=enum16{"Connect", "Read", "Write", "Close"}."Write", "error in"=w157, "Send Command"=T8 "Analyze Log", "Log Path"=w147, "IP Address"=w114) -> ("error out"=w136:errorcluster)  [unwired: 4 in, 2 out]
        n90 = call "时间延迟3"("error in (no error)"=w136, "Delay Time (s)"=1.0) -> ("error out"=w135:errorcluster)  [unwired: 9 in]
        n91 = call "Remote PC - Client_DUT1.vi"("Flow Contorl"=enum16{"Connect", "Read", "Write", "Close"}."Write", "error in"=w135, "Send Command"=T8 "Write SFC-Results", "IP Address"=w114) -> ("error out"=w141:errorcluster)  [unwired: 5 in, 2 out]
        n92 = call "时间延迟"("error in (no error)"=w141, "Delay Time (s)"=1.0) -> ("error out"=w133:errorcluster)  [unwired: 9 in]
        n93 = Merge Errors(w133, w134) -> (w132:errorcluster)
        n94 = call "Remote PC - Client_DUT2.vi"("error in"=w132, "Send Command"=T8 "Write SFC-Results", "IP Address"=w103) -> ("error out"=w139:errorcluster)  [unwired: 6 in, 2 out]
        n95 = call "时间延迟2"("error in (no error)"=w139, "Delay Time (s)"=1.0) -> ("error out"=w131:errorcluster)  [unwired: 9 in]
        n96 = call "Remote PC - Client_DUT2.vi"("Flow Contorl"=enum16{"Connect", "Read", "Write", "Close"}."Close", "error in"=w131, "IP Address"=w103) -> ("error out"=w215:errorcluster)  [unwired: 6 in, 2 out]
        n97 = call "Remote PC - Client_DUT1.vi"("Flow Contorl"=enum16{"Connect", "Read", "Write", "Close"}."Close", "error in"=w131, "IP Address"=w114) -> ("error out"=w208:errorcluster)  [unwired: 6 in, 2 out]
        n98 = Merge Errors(w208, w215) -> (w194:errorcluster)
        n99 = call "WLAN - Test - UTIL - GetTime.vi"("error in (no error)"=w194) -> ("error out"=w193:errorcluster, "millisecond timer value"=w192:u32)  [unwired: 8 in, 1 out]
      }
    }
    frame True {
      n100 = for {
        N: w411 -> [_]
        tunnel: w414 -> [w506]
        tunnel: w413 -> [w482]
        tunnel: w412 -> [w497]
        tunnel: [w489] -> w404
        tunnel: [w488] -> w407
        tunnel: w408 -> [w462]
        tunnel: w408 -> [w455]
        tunnel: w409 -> [w454]
        tunnel: w408 -> [w441]
        tunnel: w410 -> [w426]
        tunnel: [w418] -> w406
        tunnel: [w417] -> w405
        i -> [w503]
        stop <- w420 stop-if-true
        w438 = Ctl_Ant_Number."3" ("Ant Number")
        w443 = "DUT 1" ("Board Name (TX RX Verification)")
        w444 = "192.168.1.1" ("ART2 IP Address (\"\": localhost)")
        n101 = call "Pathloss Folder Path.vi"() -> ()  [unwired: 11 in, 1 out]
        n102 = call "niSwitch_ctl.vi"("Flow Control"=enum16{"Init", "1<->2", "1<->3", "Close"}."1<->2", "error in"=w506) -> ("error out"=w481:errorcluster)  [unwired: 7 in, 2 out]
        n103 = Increment(x=w503) -> (x+1=→"RUN TIMES 2":i32)
        n104 = disable-structure shown="Enabled" {
          disable-tunnel: [w574 w576] -> w501
          disable-tunnel: w481 -> [w572 w576]
          disable-tunnel: w444 -> [w571 _]
          frame Disabled {
            n105 = call "Remote PC - Client_DUT1.vi"("Remote Sever Port (2800)"=u16 1000, "Flow Contorl"=enum16{"Connect", "Read", "Write", "Close"}."Connect", "error in"=w572, "IP Address"=w571) -> ("error out"=w574:errorcluster)  [unwired: 5 in, 2 out]
          }
          frame Enabled {
          }
        }
        n106 = call "Remote PC - Client_DUT1.vi"("Flow Contorl"=enum16{"Connect", "Read", "Write", "Close"}."Write", "error in"=w501, "Send Command"=T8 "WLAN", "IP Address"=w444) -> ("error out"=w477:errorcluster)  [unwired: 5 in, 2 out]
        n107 = call "Remote PC - Client_DUT1.vi"("Flow Contorl"=enum16{"Connect", "Read", "Write", "Close"}."Write", "error in"=w477, "Send Command"=T8 "Read SFC", "IP Address"=w444) -> ("error out"=w474:errorcluster, "MAC&SN"=w436:string)  [unwired: 5 in, 1 out]
        "MAC&SN 3" <- w436
        n108 = call "Remote PC - Client_DUT1.vi"("Flow Contorl"=enum16{"Connect", "Read", "Write", "Close"}."Write", "error in"=w474, "Send Command"=T8 "Write SFC-Start to run", "IP Address"=w444) -> ("error out"=w473:errorcluster)  [unwired: 5 in, 2 out]
        n109 = call "Time Delay4"("error in (no error)"=w473, "Delay Time (s)"=3.0) -> ("error out"=w437:errorcluster)  [unwired: 9 in]
        n110 = call "Search_SN_MAC.vi"("MAC&SN"=w436) -> ("MAC"=w434:string, "SN"=w435:string)  [unwired: 9 in]
        n111 = Build Array("DUT S/N " ("string"), w435) -> (w433:string[])
        n112 = Build Array("DUT MAC" ("string"), w434) -> (w432:string[])
        n113 = Build Array(w433, w432, w426) -> (w431:string[][])
        n114 = for {
          shift-right: [w511] -> w425
          shift-left: w437 -> [w512]
          tunnel: w431 -> [w510] mode=indexing
          n115 = call "Report - Flow Control.vi"("DUT Number (Each Control)"=T5 "DUT 1", "Text Input"=w510, "error in"=w512, "Reprot Log Flow Control"=Report_Log_Flow_Control."Append Customized Text") -> ("error out"=w511:errorcluster)  [unwired: 10 in, 5 out]
        }
        n116 = call "WLAN - QCA - Test Flow Control_DUT1.vi"("RFSA In (Initial)"=w482, "RFSG In (Initial)"=w497, "error in"=w425, "NB IP (Initial)"=w444, "Function"=WLAN_Flow_Control."Initial WLAN DUT", "DUT Number (Initial, Create Log, Save Time)"=w443) -> ("RFSA Out"=w496:refnum<k15>, "RFSG Out"=w495:refnum<k15>, "error out"=w505:errorcluster)  [unwired: 10 in, 1 out]
        n117 = Unbundle By Name(w454) -> ("Calibiration?"=w419:bool)
        n118 = case shown="True" w419 {
          tunnel: w505 -> [w559 w570]
          tunnel: w496 -> [w561 w569]
          tunnel: w495 -> [w560 w568]
          tunnel: [w561 w567] -> w487
          tunnel: [w560 w566] -> w486
          tunnel: [w559 w565] -> w483
          tunnel: w443 -> [_ w564]
          tunnel: w438 -> [_ w563]
          frame False {
          }
          frame True {
            n119 = call "WLAN - QCA - Test Flow Control_DUT1.vi"("RFSA In (Initial)"=w569, "RFSG In (Initial)"=w568, "error in"=w570, "Ant Number"=w563, "Function"=WLAN_Flow_Control."Power Calibration", "DUT Number (Initial, Create Log, Save Time)"=w564) -> ("RFSA Out"=w567:refnum<k15>, "RFSG Out"=w566:refnum<k15>, "error out"=w565:errorcluster)  [unwired: 10 in, 1 out]
          }
        }
        n120 = case shown="False" FALSE {
          selector: FALSE -> [_ w581]
          tunnel: w487 -> [w579 w591]
          tunnel: w486 -> [w578 w590]
          tunnel: [w579 w589] -> w485
          tunnel: [w578 w588] -> w484
          tunnel: w443 -> [_ w587]
          tunnel: w483 -> [w577 w586]
          tunnel: w438 -> [_ w585]
          tunnel: w444 -> [_ w584]
          tunnel: w436 -> [_ w583]
          tunnel: [w577 w580] -> w424
          frame False {
          }
          frame True {
            n121 = call "WLAN - QCA - Test Flow Control_DUT1.vi"("RFSA In (Initial)"=w591, "RFSG In (Initial)"=w590, "Write Calibration"=w581, "error in"=w586, "Ant Number"=w585, "NB IP (Initial)"=w584, "Function"=WLAN_Flow_Control."Write Memory", "DUT Number (Initial, Create Log, Save Time)"=w587, "MAC&SN"=w583) -> ("RFSA Out"=w589:refnum<k15>, "RFSG Out"=w588:refnum<k15>, "error out"=w580:errorcluster)  [unwired: 7 in, 1 out]
          }
        }
        n122 = Unbundle By Name(w454) -> ("Verification?"=w453:bool)
        n123 = case shown="True" w453 {
          tunnel: "Select Test Item (TX Verification) 2" -> [_ w557]
          tunnel: [w546 w556] -> w423
          tunnel: [w545 w555] -> w494
          tunnel: [w544 w554] -> w493
          tunnel: w424 -> [w546 w553]
          tunnel: w485 -> [w545 w552]
          tunnel: w484 -> [w544 w551]
          tunnel: w462 -> [_ w550]
          tunnel: w444 -> [_ w549]
          tunnel: w443 -> [_ w548]
          tunnel: w438 -> [_ w547]
          frame False {
          }
          frame True {
            n124 = call "WLAN - QCA - Test Flow Control_DUT1.vi"("RFSA In (Initial)"=w552, "RFSG In (Initial)"=w551, "error in"=w553, "Ant Number"=w547, "Select Test Item (TX Verification)"=w557, "Stop if fail"=w550, "NB IP (Initial)"=w549, "Function"=WLAN_Flow_Control."TX Verification", "DUT Number (Initial, Create Log, Save Time)"=w548) -> ("RFSA Out"=w555:refnum<k15>, "RFSG Out"=w554:refnum<k15>, "error out"=w556:errorcluster)  [unwired: 7 in, 1 out]
          }
        }
        n125 = call "niSwitch_ctl.vi"("Flow Control"=enum16{"Init", "1<->2", "1<->3", "Close"}."1<->3", "error in"=w423) -> ("error out"=w422:errorcluster)  [unwired: 7 in, 2 out]
        n126 = case shown="True" w453 {
          tunnel: [w530 w543] -> w416
          tunnel: w494 -> [w532 w542]
          tunnel: w493 -> [w531 w541]
          tunnel: [w532 w540] -> w449
          tunnel: [w531 w539] -> w448
          tunnel: w422 -> [w530 w538]
          tunnel: w444 -> [_ w537]
          tunnel: w443 -> [_ w536]
          tunnel: w438 -> [_ w535]
          tunnel: w455 -> [_ w533]
          frame False {
          }
          frame True {
            n127 = call "WLAN - QCA - Test Flow Control_DUT1.vi"("RFSA In (Initial)"=w542, "RFSG In (Initial)"=w541, "error in"=w538, "Ant Number"=w535, "Stop if fail"=w533, "NB IP (Initial)"=w537, "Function"=WLAN_Flow_Control."RX Verification", "DUT Number (Initial, Create Log, Save Time)"=w536) -> ("RFSA Out"=w540:refnum<k15>, "RFSG Out"=w539:refnum<k15>, "error out"=w543:errorcluster)  [unwired: 8 in, 1 out]
          }
        }
        n128 = call "Report - Flow Control.vi"("error in"=w416, "Reprot Log Flow Control"=Report_Log_Flow_Control."Read Log File") -> ("Cluster 2"=w451:T2, "error out"=w428:errorcluster)  [unwired: 12 in, 4 out]
        "Results 2" <- w451
        n129 = Unbundle By Name(w451) -> ("DUT1 p/f"=w442:bool, "DUT2 p/f"=w440:bool)
        n130 = And(x=w441, y=w440) -> ()  [unwired: 1 out]
        n131 = And(x=w441, y=w442) -> (x .and. y?=w439:bool)
        n132 = case shown="True" w439 {
          selector: w439 -> [_ w520]
          tunnel: w449 -> [w517 w529]
          tunnel: w448 -> [w516 w528]
          tunnel: [w517 w527] -> w447
          tunnel: [w516 w526] -> w446
          tunnel: w416 -> [w515 w525]
          tunnel: [w515 w524] -> w445
          tunnel: w444 -> [_ w523]
          tunnel: w443 -> [_ w522]
          tunnel: w438 -> [_ w519]
          tunnel: w436 -> [_ w518]
          frame False {
          }
          frame True {
            n133 = call "WLAN - QCA - Test Flow Control_DUT1.vi"("RFSA In (Initial)"=w529, "RFSG In (Initial)"=w528, "Write Calibration"=w520, "error in"=w525, "Ant Number"=w519, "NB IP (Initial)"=w523, "Function"=WLAN_Flow_Control."Write Memory", "DUT Number (Initial, Create Log, Save Time)"=w522, "MAC&SN"=w518) -> ("RFSA Out"=w527:refnum<k15>, "RFSG Out"=w526:refnum<k15>, "error out"=w524:errorcluster)  [unwired: 7 in, 1 out]
          }
        }
        n134 = call "WLAN - QCA - Test Flow Control_DUT1.vi"("RFSA In (Initial)"=w447, "RFSG In (Initial)"=w446, "error in"=w445, "NB IP (Initial)"=w444, "Function"=WLAN_Flow_Control."Close WLAN Test") -> ("RFSA Out"=w418:refnum<k15>, "RFSG Out"=w417:refnum<k15>, "error out"=w429:errorcluster)  [unwired: 11 in, 1 out]
        n135 = Merge Errors(w429, w428) -> (w491:errorcluster)
        n136 = call "niSwitch_ctl.vi"("Flow Control"=enum16{"Init", "1<->2", "1<->3", "Close"}."Close", "error in"=w491) -> ("error out"=w490:errorcluster)  [unwired: 7 in, 2 out]
        n137 = local read "DUT1 log path"() -> (w415:path)
        n138 = call "Remote PC - Client_DUT1.vi"("Flow Contorl"=enum16{"Connect", "Read", "Write", "Close"}."Write", "error in"=w490, "Send Command"=T8 "KILLWLAN", "IP Address"=w444) -> ("error out"=w469:errorcluster)  [unwired: 5 in, 2 out]
        n139 = call "Remote PC - Client_DUT1.vi"("Flow Contorl"=enum16{"Connect", "Read", "Write", "Close"}."Write", "error in"=w469, "Send Command"=T8 "Send Log", "Log Path"=w415, "IP Address"=w444) -> ("error out"=w468:errorcluster)  [unwired: 4 in, 2 out]
        n140 = call "Remote PC - Client_DUT1.vi"("Flow Contorl"=enum16{"Connect", "Read", "Write", "Close"}."Write", "error in"=w468, "Send Command"=T8 "Analyze Log", "Log Path"=w415, "IP Address"=w444) -> ("error out"=w458:errorcluster)  [unwired: 4 in, 2 out]
        n141 = call "时间延迟6"("error in (no error)"=w458, "Delay Time (s)"=1.0) -> ("error out"=w457:errorcluster)  [unwired: 9 in]
        n142 = call "Remote PC - Client_DUT1.vi"("Flow Contorl"=enum16{"Connect", "Read", "Write", "Close"}."Write", "error in"=w457, "Send Command"=T8 "Write SFC-Results", "Log Path"=w415, "IP Address"=w444) -> ("error out"=w461:errorcluster)  [unwired: 4 in, 2 out]
        n143 = call "时间延迟4"("error in (no error)"=w461, "Delay Time (s)"=1.0) -> ("error out"=w421:errorcluster)  [unwired: 9 in]
        n144 = call "Remote PC - Client_DUT1.vi"("Flow Contorl"=enum16{"Connect", "Read", "Write", "Close"}."Close", "error in"=w421, "IP Address"=w444) -> ("error out"=w420:errorcluster)  [unwired: 6 in, 2 out]
        n145 = call "WLAN - Test - UTIL - GetTime.vi"("error in (no error)"=w420) -> ("error out"=w489:errorcluster, "millisecond timer value"=w488:u32)  [unwired: 8 in, 1 out]
      }
    }
  }
  n146 = Subtract(x=w35, y=w32) -> (x-y=w33:u32)
  n147 = Divide(x=w33, y=1000.0) -> (x/y=→"Total test time":dbl)
  n148 = call <instrlib>:"niRFSA Close.vi"("instrument handle"=w2, "error in"=w5) -> ("error out"=w18:errorcluster)  [unwired: 13 in]
  n149 = call <instrlib>:"niRFSG Close.vi"("instrument handle"=w36, "error in"=w5) -> ("error out"=w17:errorcluster)  [unwired: 13 in]
  n150 = Merge Errors(w18, w17, w5) -> (w7:errorcluster)
  n151 = call <vilib>:"Simple Error Handler.vi"("error in (no error)"=w7) -> ()  [unwired: 4 in, 5 out]
